vi "Build AFM Litho Installer.vi"() -> ()   [LabVIEW 2019]
uses:
  <vilib>/AppBuilder/AB_API_Simple/Build Specification Version.ctl
  <vilib>/AppBuilder/AB_API_Simple/Set Build Specification Version (path).vi
  <vilib>/AppBuilder/AB_API_Simple/Build (path).vi
  <vilib>/AppBuilder/AB_API_Simple/NI_App_Builder_API.lvlib
  <vilib>/MakerHub/Toolbox/LMH-Toolbox.lvlib
  <userlib>/LevyLab/Build Support/PostBuildSupport/PostBuildSupport.lvclass
panel:
  in  "Version (maj.min.fix.build)":string="10.1.0.1"
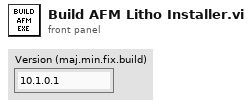
[diagram p1: front panel]
types:
  T1 = typedef "NI_App_Builder_API.lvlib/Build Specification Version.ctl" = cluster{"Major":u16, "Minor":u16, "Fix":u16, "Build":u16}
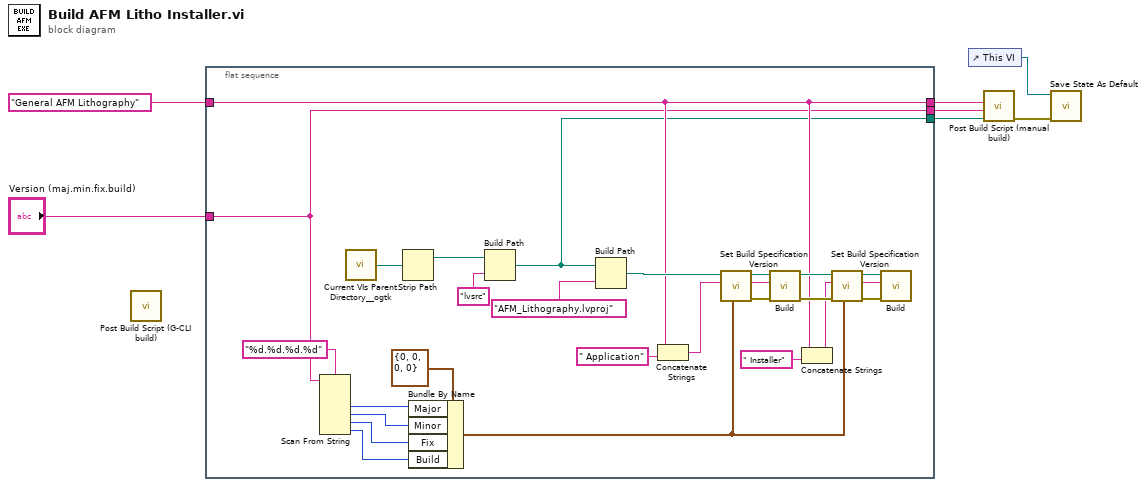
[diagram p0: block diagram]
diagram:
  n1 = call <userlib>:"Post Build Script (G-CLI build).vi"() -> ()  [unwired: 11 in, 1 out]
  n2 = flat-sequence {
    tunnel: "General AFM Lithography" ("Name of build specification") -> [w10]
    tunnel: "Version (maj.min.fix.build)" -> [w9]
    tunnel: [w10] -> w1
    tunnel: [w9] -> w2
    tunnel: [w8] -> w4
    frame #0 {
      n3 = Scan From String(format string="%d.%d.%d.%d", input string=w9) -> (output 1=w21:i32, output 2=w20:i32, output 3=w19:i32, output 4=w18:i32)  [unwired: 6 in, 3 out]
      n4 = call <userlib>:"Current VIs Parent Directory__ogtk.vi"() -> ("Parent Directory (+ Relative)"=w29:path)  [unwired: 5 in]
      n5 = Strip Path(path=w29) -> (stripped path=w28:path)  [unwired: 1 out]
      n6 = Bundle By Name(cluster=T1 {"Major"=0, "Minor"=0, "Fix"=0, "Build"=0} ("Build Specification Version"), "Major"=w21, "Minor"=w20, "Fix"=w19, "Build"=w18) -> (w17:T1)
      n7 = Build Path(base path=w28, name or relative path="lvsrc") -> (appended path=w8:path)
      n8 = Build Path(base path=w8, name or relative path="AFM_Lithography.lvproj") -> (appended path=w13:path)
      n9 = Concatenate Strings(w10, " Application" ("string")) -> (w11:string)
      n10 = call-poly <vilib>:"Set Build Specification Version.vi"("Build Specification Version"=w17, "Name of build specification"=w11, "Path to project"=w13) -> ("error out"=w26:errorcluster)  [unwired: 8 in]
      n11 = call-poly <vilib>:"Build.vi"("error in (no error)"=w26, "Name of build specification (if empty: build all)"=w11, "Path to project"=w13) -> ("error out"=w24:errorcluster)  [unwired: 7 in, 1 out]
      n12 = Concatenate Strings(w10, " Installer" ("string")) -> (w12:string)
      n13 = call-poly <vilib>:"Set Build Specification Version.vi"("Build Specification Version"=w17, "error in (no error)"=w24, "Name of build specification"=w12, "Path to project"=w13) -> ("error out"=w25:errorcluster)  [unwired: 7 in]
      n14 = call-poly <vilib>:"Build.vi"("error in (no error)"=w25, "Name of build specification (if empty: build all)"=w12, "Path to project"=w13) -> ()  [unwired: 7 in, 2 out]
    }
  }
  n15 = control-ref of="This VI"() -> (w5:refnum<vi>)
  n16 = call <userlib>:"Post Build Script (manual build).vi"("Package Source Folder"=w4, "Package Version"=w2, "Product Name"=w1) -> ("error out"=w3:errorcluster)  [unwired: 8 in]
  n17 = call <vilib>:"Save State As Default.vi"("Error In"=w3, "Target VI"=w5) -> ()  [unwired: 8 in, 2 out]
